vi "MachineSimulator.vi"() -> ()   [LabVIEW 2014]
panel:
  in  "Color":u32(colorbox)
  in  "BeamLoc":cluster{"X":dbl, "Y":dbl}={"X"=250.0, "Y"=250.0} {"X" min=-250.0 max=250.0; "Y" min=-250.0 max=250.0}
  in  "stop":bool
  out "Pic":picture
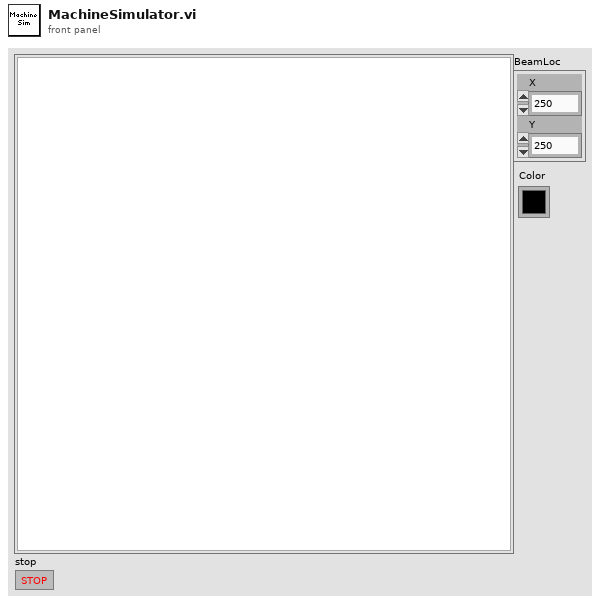
[diagram p1: front panel]
types:
  T1 = cluster{"Width":u16, "Style":enum32{"Solid", "Dash", "Dot", "DashDot", "DashDotDot"}}
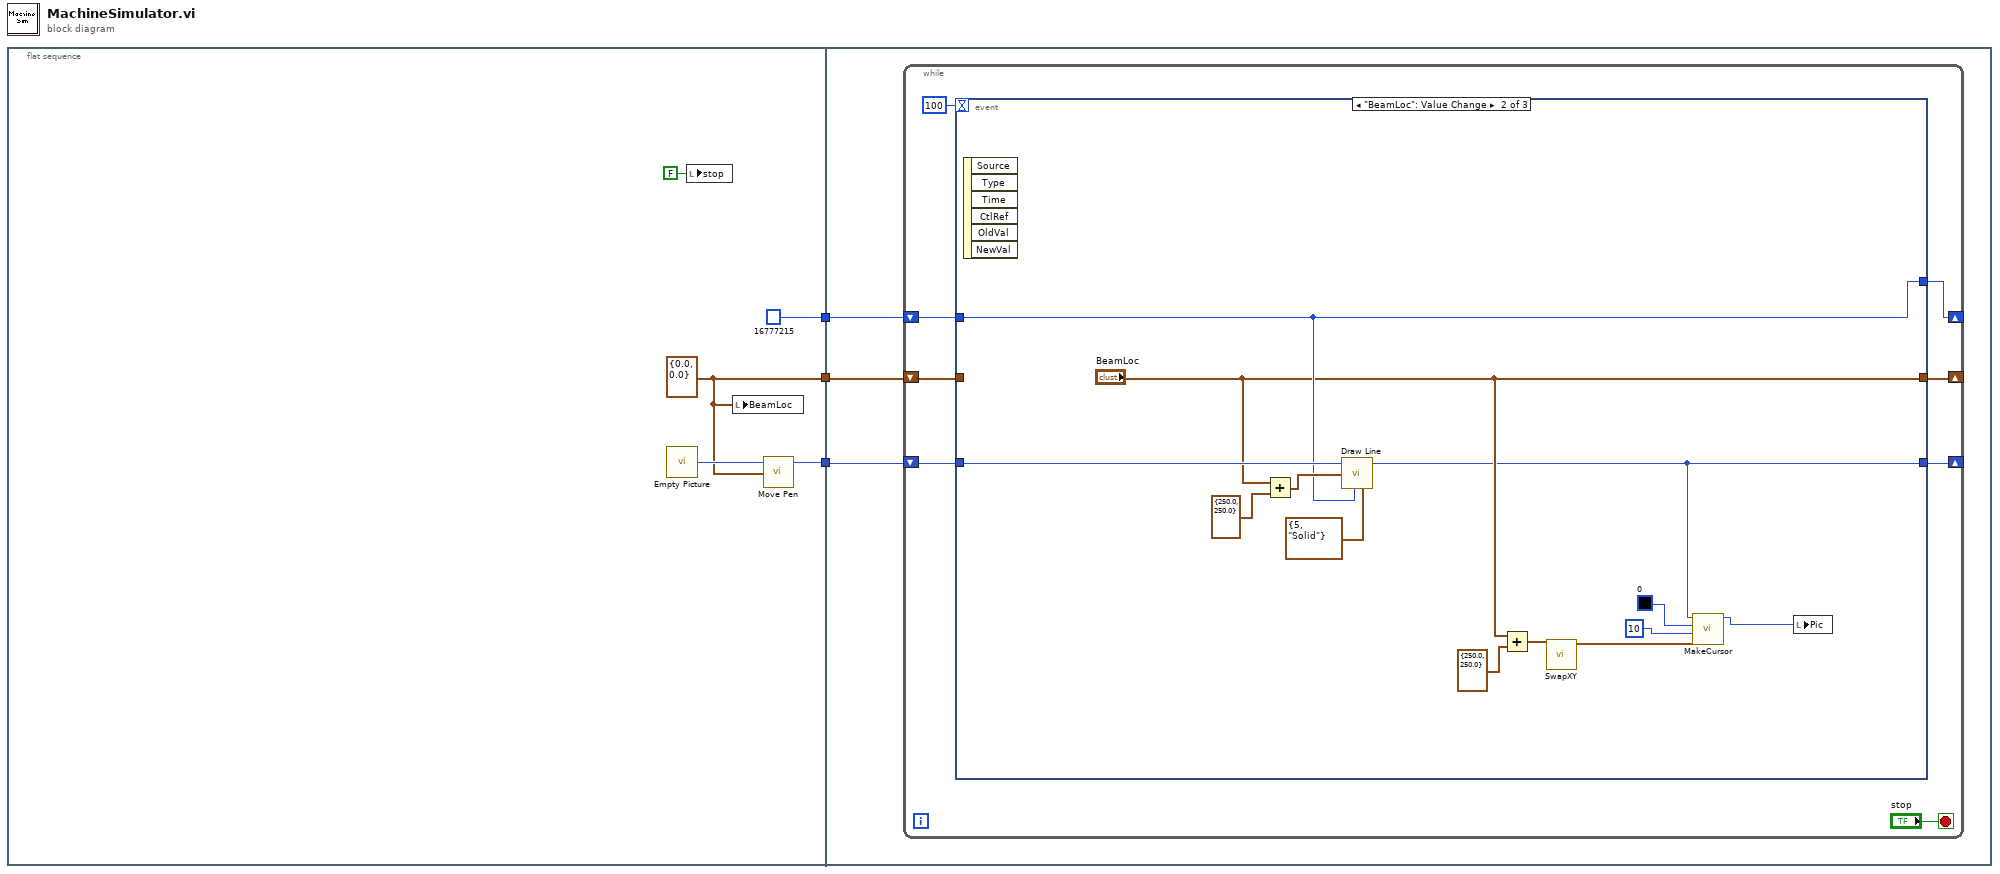
[diagram p0: block diagram]
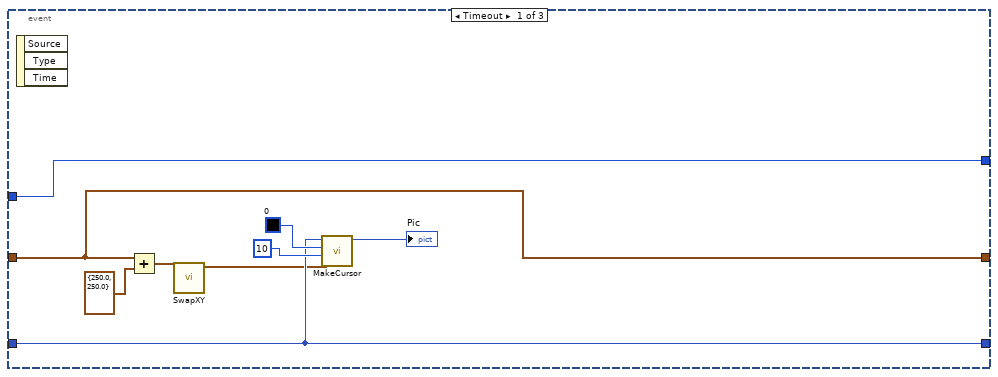
[diagram p2: hidden frame]
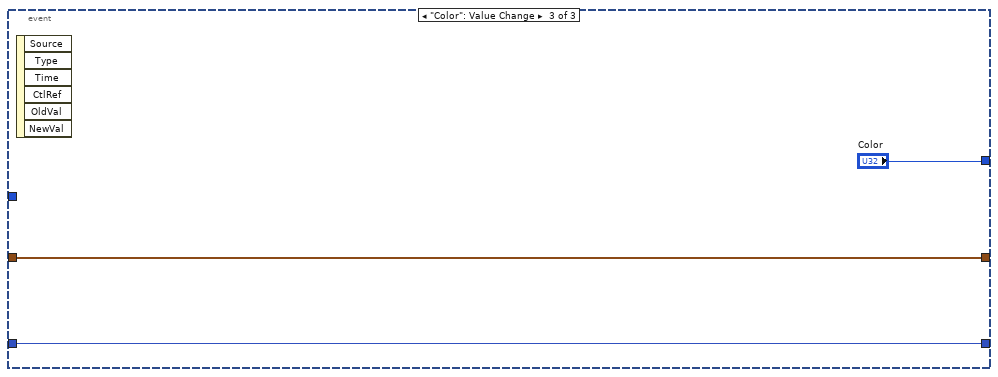
[diagram p3: hidden frame]
diagram:
  n1 = flat-sequence {
    tunnel: [u32 16777215] -> w3
    tunnel: [w5] -> w2
    tunnel: [w7] -> w1
    tunnel: w3 -> [w11]
    tunnel: w2 -> [w10]
    tunnel: w1 -> [w9]
    frame #0 {
      w5 = cluster{"X":dbl, "Y":dbl} {"X"=0.0, "Y"=0.0}
      n2 = call "Empty Picture"() -> ("empty picture"=w6:picture)
      n3 = local write "stop"(FALSE ("stop")) -> ()
      n4 = local write "BeamLoc"(w5) -> ()
      n5 = call <vilib>:"Move Pen.vi"("new position"=w5, "picture"=w6) -> ("new picture"=w7:picture)  [unwired: 3 in]
    }
    frame #1 {
      n6 = while {
        shift-right: [w13] -> _
        shift-left: w11 -> [w12]
        shift-right: [w14] -> _
        shift-left: w10 -> [w17]
        shift-right: [w15] -> _
        shift-left: w9 -> [w16]
        stop <- "stop" stop-if-true
        n7 = event shown="[1] \"BeamLoc\": Value Change" {
          selector: _ -> [_ _ _]
          dyn-events: _ -> [_ _ _]
          timeout: 100 -> [_ _ _]
          tunnel: w17 -> [w23 _ w43]
          tunnel: w16 -> [w25 w41 w42]
          tunnel: [w25 w30 w42] -> w15
          tunnel: [w23 "BeamLoc" w43] -> w14
          tunnel: [w22 w38 "Color"] -> w13
          tunnel: w12 -> [w22 w38 _]
          event Timeout {
            n8 = event-data() -> ()  [unwired: 1 in, 3 out]
            n9 = Add(x=w23, y=cluster{"X":dbl, "Y":dbl} {"X"=250.0, "Y"=250.0}) -> (x+y=w21:cluster{"X":dbl, "Y":dbl})
            n10 = call "SwapXY.vi"("Point"=w21) -> ("Swapped"=w20:cluster{"X Cen":sgl, "Y Cen":sgl})  [unwired: 10 in]
            n11 = call "MakeCursor.vi"("WindowLoc"=w20, "Size"=u8 10, "Color"=u32 0, "PicIn"=w25) -> ("CursorOut"=→"Pic":picture)  [unwired: 7 in]
          }
          event "BeamLoc": Value Change {
            n12 = event-data() -> ()  [unwired: 1 in, 6 out]
            n13 = Add(x="BeamLoc", y=cluster{"X":dbl, "Y":dbl} {"X"=250.0, "Y"=250.0}) -> (x+y=w39:cluster{"X":dbl, "Y":dbl})
            n14 = call <vilib>:"Draw Line.vi"("picture"=w41, "end point"=w39, "color(black)"=w38, "pen"=T1 {"Width"=5, "Style"=enum."Solid"}) -> ("new picture"=w30:picture)  [unwired: 5 in]
            n15 = Add(x="BeamLoc", y=cluster{"X":dbl, "Y":dbl} {"X"=250.0, "Y"=250.0}) -> (x+y=w33:cluster{"X":dbl, "Y":dbl})
            n16 = call "SwapXY.vi"("Point"=w33) -> ("Swapped"=w32:cluster{"X Cen":sgl, "Y Cen":sgl})  [unwired: 10 in]
            n17 = call "MakeCursor.vi"("WindowLoc"=w32, "Size"=u8 10, "Color"=u32 0, "PicIn"=w30) -> ("CursorOut"=w29:picture)  [unwired: 7 in]
            n18 = local write "Pic"(w29) -> ()
          }
          event "Color": Value Change {
            n19 = event-data() -> ()  [unwired: 1 in, 6 out]
          }
        }
      }
    }
  }
